vi "ErrorHandler.vi"   [LabVIEW 2011, in "Konvolucio MCAN120803.lvlib"]
uses:
  <instrlib>/Konvolucio MCAN120803/Konvolucio MCAN120803.lvlib
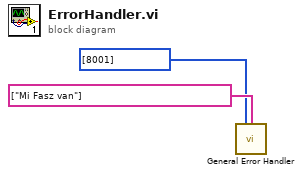
[diagram p0: block diagram]
diagram:
  n1 = call <vilib>:"General Error Handler.vi"("[user-defined codes]"=i32[] [8001], "[user-defined descriptions]"=string[] ["Mi Fasz van"]) -> ()  [unwired: 9 in, 5 out]
